vi "CopyArrayToImageGreyscale.vi"(8 "error in (no error)":errorcluster, 10 "Greyscale Destination Image":refnum<data-value>, 11 "Source":u8[][](array[numeric])) -> (0 "error out":errorcluster, 3 "Greyscale Destination Image (duplicate)":refnum<data-value>)   [LabVIEW 2020, in "g_ar_toolkit.image.lvlib"]
uses:
  g_ar_toolkit.image.lvlib
  26c70cee-9332-41f4-9755-08948a885cbe.vi
  bin/g_ar_toolkit.1.32.dll
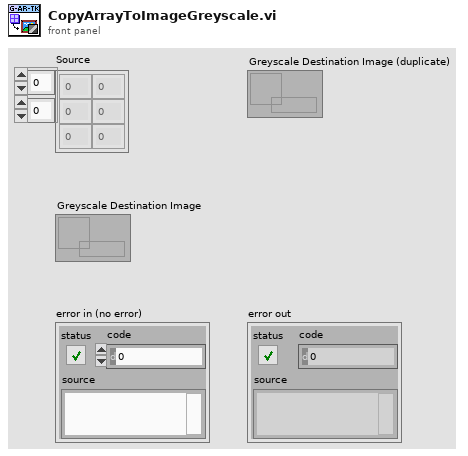
[diagram p1: front panel]
types:
  T1 = typedef "g_ar_toolkit_common.lvlib/Image Size (Integer).ctl" = cluster{"Width":u16, "Height":u16}
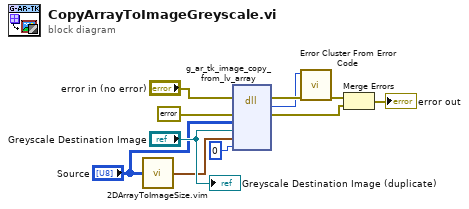
[diagram p0: block diagram]
diagram:
  n1 = call "2DArrayToImageSize.vim"("Array"="Source") -> ("Image Size"=w5:T1)
  n2 = dll-call lib="C:/serenial/libraries/g-augmented-reality-toolkit/LabVIEW/bin/g_ar_toolkit.1.*.*" fn="g_ar_tk_image_copy_from_lv_array" ("g_ar_toolkit.*.*:g_ar_tk_image_copy_from_raw_memory")(error in="error in (no error)", "error_cluster"=errorcluster {"status"=FALSE, "code"=0, "source"=""} ("error constant"), "Source"="Source", "EDVR Dst"="Greyscale Destination Image", "Size"=w5, "third dim size"=u8 0) -> (error out=w3:errorcluster, "MgErr"=w2:i32, "error_cluster"=w10:errorcluster)  [unwired: 6 in, 1 out]
  n3 = call <vilib>:"Error Cluster From Error Code.vi"("error in (no error)"=w3, "error code (0)"=w2) -> ("error out"=w4:errorcluster)  [unwired: 7 in]
  n4 = Merge Errors(w4, w10) -> (→"error out":errorcluster)
  "Greyscale Destination Image (duplicate)" <- "Greyscale Destination Image"
